vi "InitArm.vi"   [LabVIEW 2015]
uses:
  <vilib>/Rock Robotics/WPI/CAN/TalonSRX/WPI_CANTalonSRX_APIControlMode.ctl
  <vilib>/Rock Robotics/WPI/CAN/TalonSRX/WPI_CANTalonSRX_APIFeedbackSelect.ctl
  <vilib>/Rock Robotics/WPI/MotorControl/WPI_MotorControlOpenCANTalonSRX.vi
types:
  T1 = typedef "WPI_CANTalonSRX_APIFeedbackSelect.ctl" = enum16{"Digital Quadrature Encoder", "Analog Potentiometer", "Analog Encoder", "Count on Quad-A (Rising-Edge)", "Count on Quad-A (Falling-Edge)", "CTR Magnetic Enc (Absolute)", "CTR Magnetic Enc (Relative)", "Pulse Width"}
  T2 = typedef "WPI_CANTalonSRX_APIControlMode.ctl" = enum8{"Percent VBus", "Speed", "Position", "Slave", "Unchanged / Invalid", "Voltage Compensation", "Current", "Motion Profile"}
  T3 = typedef "constants.ctl" = cluster{"motorConstants":cluster{"leftDriveMotor":u8, "rightDriveMotor":u8, "climberWinch":T4, "shooterTopFlyWheel":T4, "shooterBottomFlyWheel":T4, "climberExtender":T4, "shooterIntakeWheel":u8, "Front Arm Motor":u8}, "arduinoInputChannel":cluster{"armAngleUp":i32, "intakeWheelSpinIn":i32, "winchUp":i32, "extenderUp":i32, "AimingAuto":i32, "extenderDown":i32, "FrontArmAxis":i32, "shooter up/down":i32}, "driveConstants":cluster{"firstIntervalPercent":dbl, "secondIntervalPercent":dbl, "thirdIntervalPercent":dbl}, "cRioInputChanels":cluster{"photoEye":i32, "limitExtender":i32}, "pneumaticsChannels":cluster{"angleSolenoid":T5, "shooterAnglerPneumaticForward":T5, "shooterAnglerPneumaticReverse":T5, "Pneumatics Control Module":u8}, "flyWheelConstants":cluster{"manualTopWheel":dbl, "manualBottomWheel":dbl, "autoFuncConst1":dbl, "autoFuncConst2":dbl, "autoFuncConst3":dbl, "autoFuncConst4":dbl, "Array":dbl[][]}}
  T4 = typedef "FPGA_DIOPWMChannel.ctl" = enum8{"PWM 0", "PWM 1", "PWM 2", "PWM 3", "PWM 4", "PWM 5", "PWM 6", "PWM 7", "PWM 8", "PWM 9", "PWM MXP 0", "PWM MXP 1", "PWM MXP 2", "PWM MXP 3", "PWM MXP 4", "PWM MXP 5", "PWM MXP 6", "PWM MXP 7", "PWM MXP 8", "PWM MXP 9", "Invalid"}
  T5 = typedef "WPI_SolenoidChannel.ctl" = enum8{"Solenoid 0", "Solenoid 1", "Solenoid 2", "Solenoid 3", "Solenoid 4", "Solenoid 5", "Solenoid 6", "Solenoid 7", "Invalid"}
  T6 = typedef "WPI_MotorControlDeviceRef.ctl" = cluster{"DeviceStatus":errorcluster, "Type":T7, "PWM":cluster{"PWM Channel":T4, "DeadBand":T8}, "CAN":cluster{"Device Number":u8, "Control Mode":T9, "Semaphore":T10, "Max Vout":dbl, "TalonSRX Control Mode":T2}, "Invert":bool}
  T7 = typedef "WPI_MotorControlType.ctl" = enum16{"PWM", "CAN", "CANTalonSRX"}
  T8 = typedef "WPI_PWMDeadband.ctl" = cluster{"Name":string, "maxPositivePwm":i32, "minPositivePwm":i32, "centerPwm":i32, "maxNegativePwm":i32, "minNegativePwm":i32, "angularRange":u16}
  T9 = typedef "WPI_CANJaguar_ControlMode.ctl" = enum8{"Percent VBus", "Current", "Speed", "Position", "Voltage"}
  T10 = typedef "Semaphore RefNum" = refnum<k1>
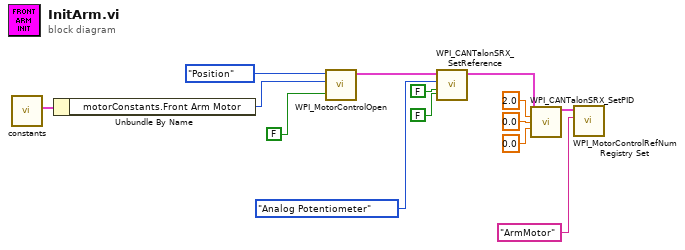
[diagram p0: block diagram]
diagram:
  n1 = call "constants.vi"() -> (2:w5:T3)  [unwired: 11 in]
  n2 = Unbundle By Name(w5) -> ("motorConstants.Front Arm Motor"=w4:u8)
  n3 = call-poly <vilib>:"WPI_MotorControlOpen.vi"("Invert"=FALSE, "Device Number"=w4, "Control Mode"=WPI_CANTalonSRX_APIControlMode."Position") -> ("MotorControlDeviceRef"=w8:T6)  [unwired: 7 in, 1 out]
  n4 = call <vilib>:"WPI_CANTalonSRX_SetReference.vi"("Reverse Closed-Loop Output"=FALSE, "Reverse Feedback Sensor"=FALSE, "Feedback Reference"=WPI_CANTalonSRX_APIFeedbackSelect."Analog Potentiometer", "CAN Talon SRX Ref"=w8) -> ("CAN Talon SRX Ref"=w9:T6)  [unwired: 6 in, 1 out]
  n5 = call <vilib>:"WPI_CANTalonSRX_SetPID.vi"("CAN Talon SRX Ref"=w9, "P"=2.0, "I"=0.0, "D"=0.0) -> ("CAN Talon SRX Ref"=w11:T6)  [unwired: 10 in, 1 out]
  n6 = call <vilib>:"WPI_MotorControlRefNum Registry Set.vi"("refnum name"="ArmMotor", "MotorControlDevRef"=w11) -> ()  [unwired: 8 in, 2 out]
